vi "Create Credit Statement from CSV.vi"(8 "error in (no error)":errorcluster, 11 "CSV Entries":string[](array[string])) -> (0 "error out":errorcluster, 3 "Statement.lvclass":refnum<class "Statement.lvclass">)   [LabVIEW 2018, in "Statement.lvclass"]
uses:
  Statement/Statement.lvclass
  Statement/Statement.lvclass/Statement.ctl
  Credit Record/Credit Transaction.lvclass
  C:/Users/jtipps/Documents/Filthy-Lucre-Budgetizer/source/support/classes/Transaction/Transaction.lvclass
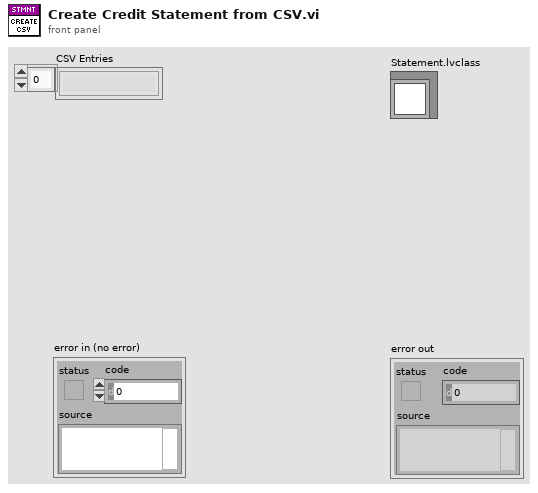
[diagram p1: front panel]
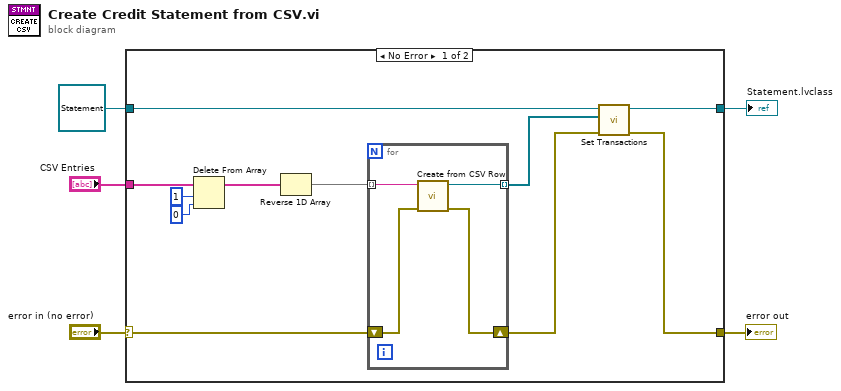
[diagram p0: block diagram]
diagram:
  n1 = case shown="No Error" "error in (no error)" {
    selector: "error in (no error)" -> [w14 w22]
    tunnel: [w12 w22] -> w4
    tunnel: [w15 w21] -> w1
    tunnel: refnum<class "Statement.lvclass"> refnum ("Statement.lvclass") -> [w16 w21]
    tunnel: "CSV Entries" -> [w8 _]
    frame No Error {
      n2 = Delete From Array(array=w8, length=1, index=0) -> (array with subset deleted=w7:string[])  [unwired: 1 out]
      n3 = Reverse 1D Array(array=w7) -> (reversed array=w6:string[])
      n4 = for {
        shift-right: [w18] -> w13
        shift-left: w14 -> [w19]
        tunnel: w6 -> [w20] mode=indexing
        tunnel: [w17] -> w11 mode=indexing
        n5 = call "Create from CSV Row.vi"("error in (no error)"=w19, "CSV Row"=w20) -> ("error out"=w18:errorcluster, "Credit Record out"=w17:refnum<class "Credit Transaction.lvclass">)  [unwired: 8 in]
      }
      n6 = call "Set Transactions.vi"("error in (no error)"=w13, "Transactions"=w11, "Statement in"=w16) -> ("error out"=w12:errorcluster, "Statement out"=w15:refnum<class "Statement.lvclass">)  [unwired: 7 in]
    }
    frame Error {
    }
  }
  "error out" <- w4
  "Statement.lvclass" <- w1
